vi "Мажор +++.vi"() -> ()   [LabVIEW 2017]
panel:
  in  "Задержка, мс":u32(knob) scale=0.0..10000.0
  in  "?":bool
  in  "Запуск программы":bool
  out "String":string
  in  "Искуственный ввод ошибки":T1(tab)
  in  "Номер элемента со второй ошибкой":i32
  in  "Номер элемента с первой ошибкой":i32
  in  "Номер элемента с третьей ошибкой":i32
  in  "Первый пакет с ошибкой":i32
  in  "Второй пакет с ошибкой":i32
  out "Первый элемент с ошибкой":i32
  out "Второй элемент с ошибкой":i32=16
  out "Третий элемент с ошибкой":i32
  out "Ошибка":bool
  out "Количество  ошибок":i32
  out "Сообщение выдаваемое получателю":dbl[](array[numeric])
  out "Сообщение на выходе канала":dbl[](array[numeric])
  out "2-х массив передаваемых данных":dbl[][](array[numeric])
  out "Массив данных поступающий в канал связи":dbl[](array[numeric])
  in  "Количество передаваемых копий":i32=5
  out "Сообщение источника":dbl[](array[numeric])
  in  "Количество генерируемых данных":i32=16
  # "Мажоритарное резервирование"
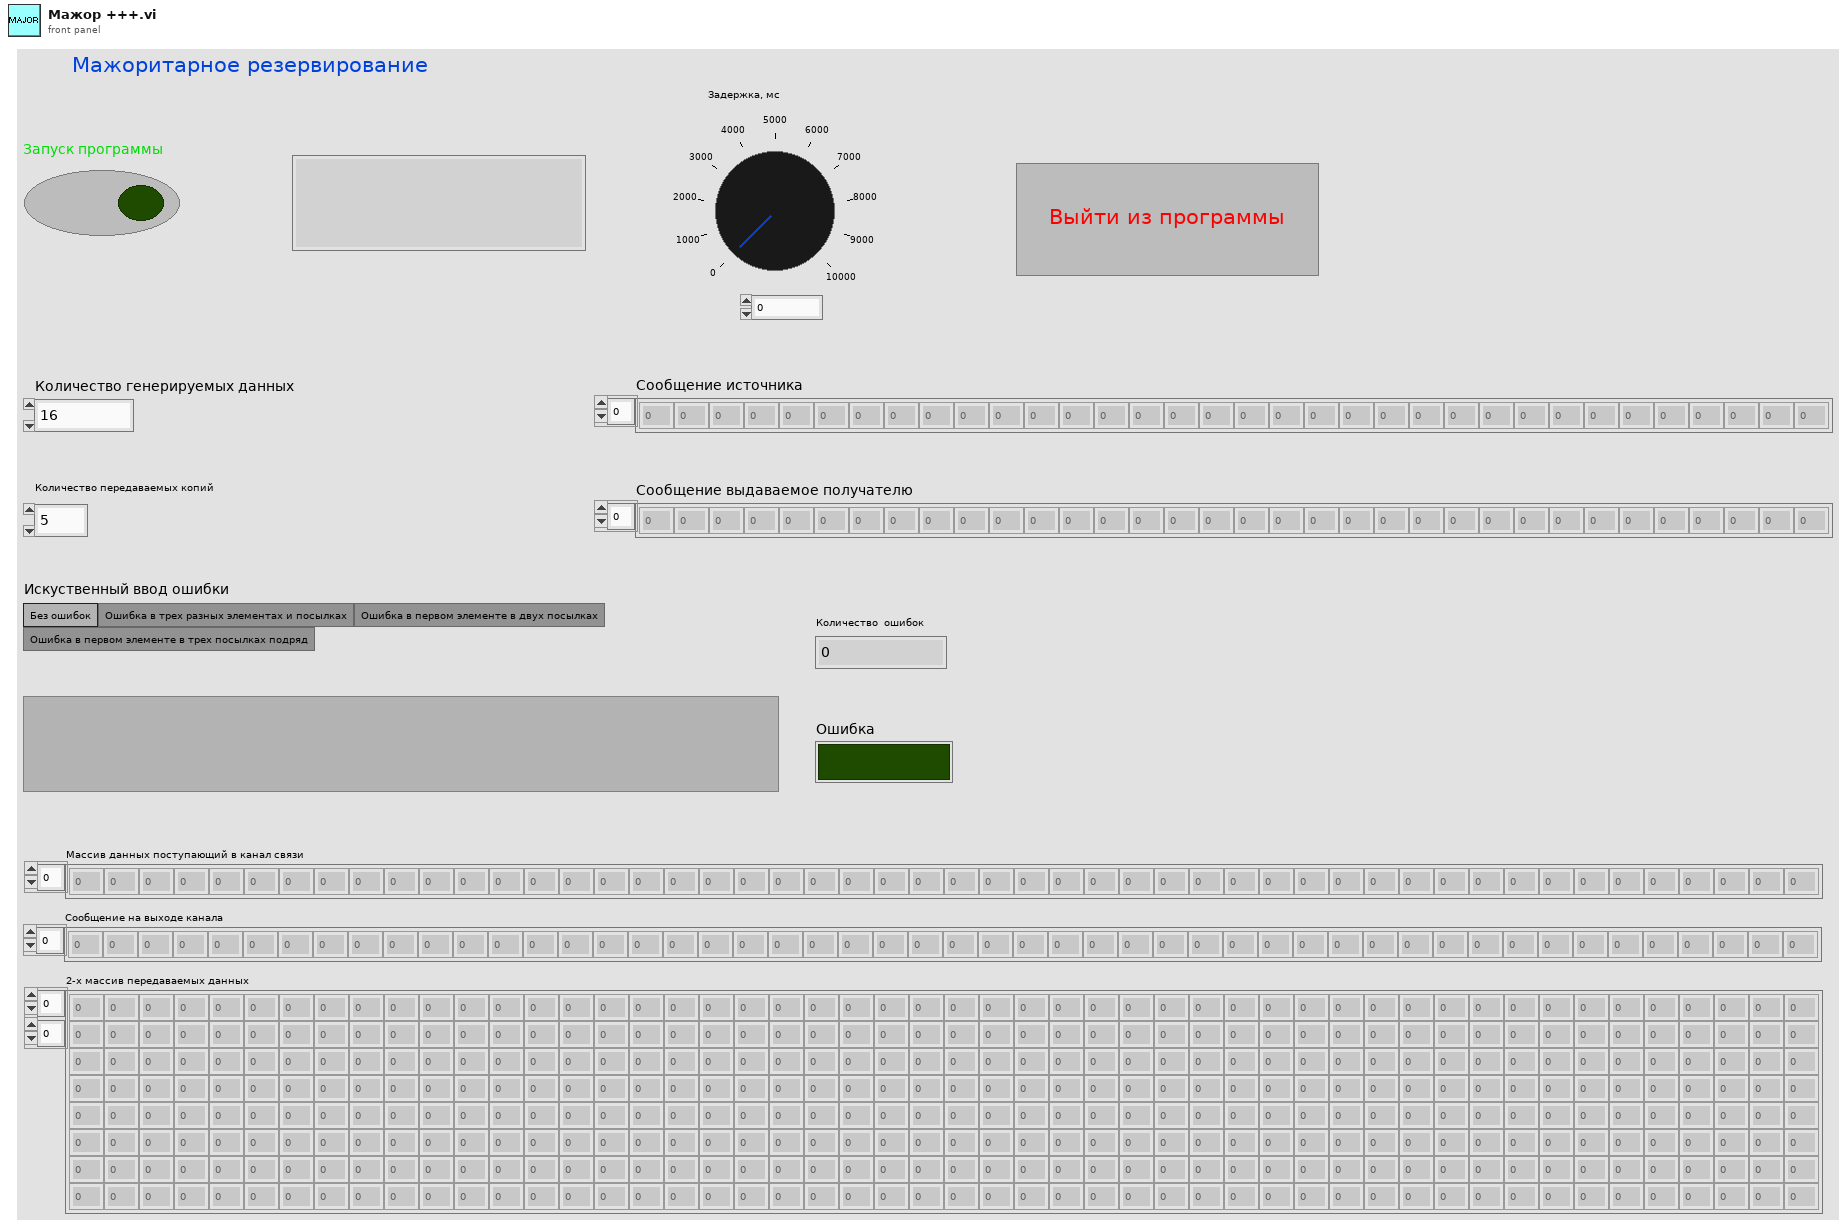
[diagram p1: front panel]
types:
  T1 = enum32{"Без ошибок", "Ошибка в трех разных элементах и посылках", "Ошибка в первом элементе в двух посылках", "Ошибка в первом элементе в трех посылках подряд"}
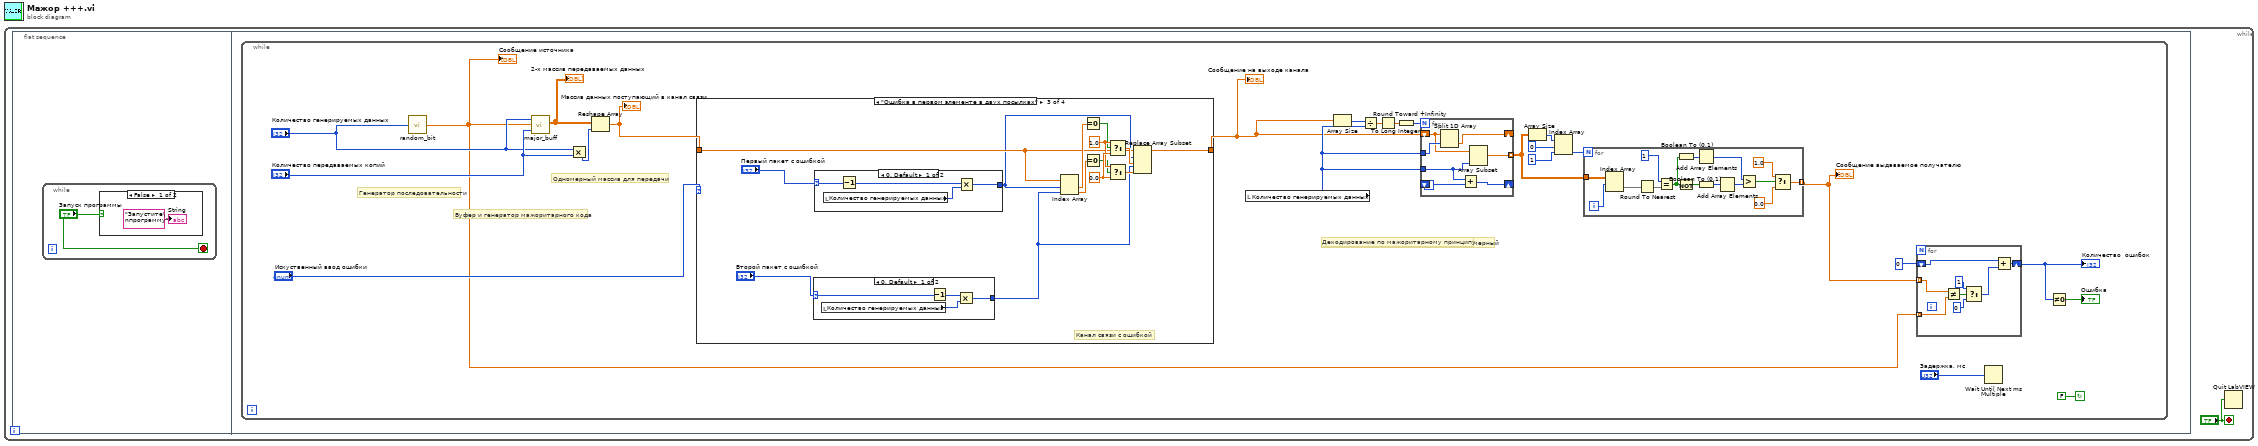
[diagram p0: block diagram]
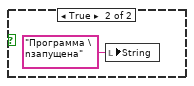
[diagram p2: hidden frame]
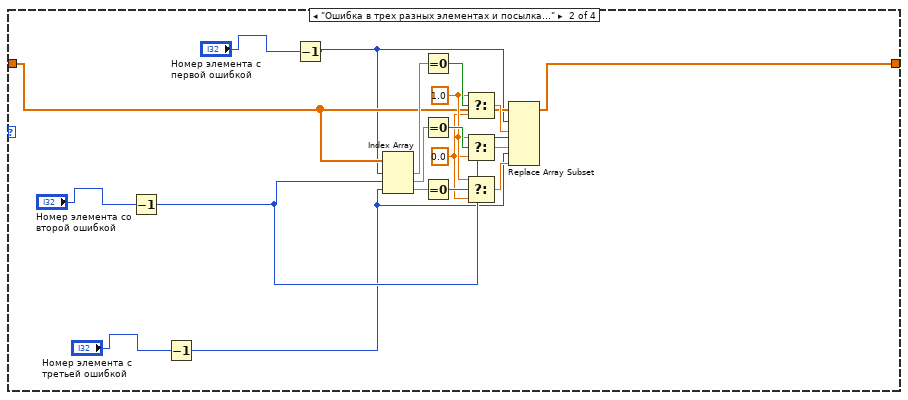
[diagram p4: hidden frame]
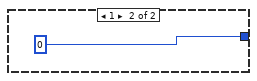
[diagram p5: hidden frame]
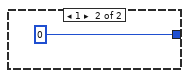
[diagram p6: hidden frame]
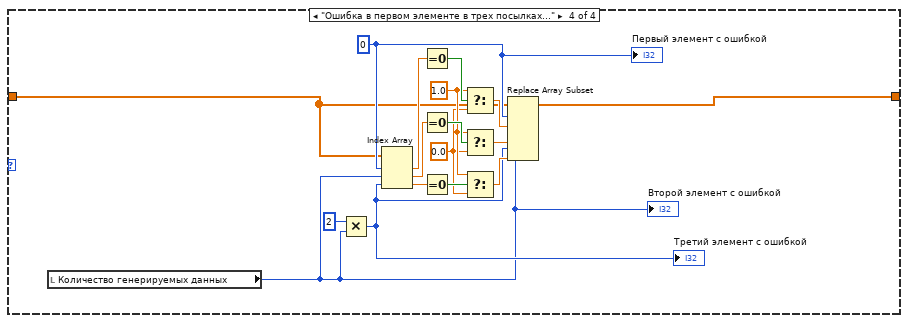
[diagram p7: hidden frame]
diagram:
  n1 = while {
    stop <- "?" stop-if-true
    n2 = flat-sequence {
      frame #0 {
        n3 = while {
          stop <- "Запуск программы" stop-if-true
          n4 = case shown="False" "Запуск программы" {
            frame False {
              "String" <- "Запустите\nпрограмму"
            }
            frame True {
              n5 = local write "String"("Программа \nзапущена") -> ()
            }
          }
        }
      }
      frame #1 {
        n6 = while {
          stop <- FALSE continue-if-true
          # "Канал связи с ошибкой"
          # "Одномерный массив для передачи"
          # "Преобразование одномерного массива в двумерный"
          # "Декодирование по мажоритарному принципу"
          # "Буфер и генератор мажоритарного кода"
          # "Генератор последовательности"
          n7 = call "random_bit.vi"("Количество бит"="Количество генерируемых данных") -> ("Биты на выходе 1"=w14:dbl[])
          "Сообщение источника" <- w14
          n8 = call "major_buff.vi"("Кол-во копий"="Количество передаваемых копий", "Размер окна"="Количество генерируемых данных", "Биты на выходе 1"=w14) -> ("Подготовленный к отправке мажоритарный код"=w17:dbl[][])  [unwired: 1 out]
          "2-х массив передаваемых данных" <- w17
          n9 = Multiply(x="Количество генерируемых данных", y="Количество передаваемых копий") -> (x*y=w25:i32)
          n10 = Reshape Array(w17, w25) -> (w11:dbl[])
          "Массив данных поступающий в канал связи" <- w11
          n11 = case shown="\"Ошибка в первом элементе в двух посылках\"" "Искуственный ввод ошибки" {
            tunnel: w11 -> [w44 w52 w69 w89]
            tunnel: [w44 w51 w68 w88] -> w10
            frame "Без ошибок", Default {
            }
            frame "Ошибка в трех разных элементах и посылках" {
              w57 = 1.0
              w56 = 0.0
              n12 = Decrement(x="Номер элемента со второй ошибкой") -> (x-1=w47:i32)
              n13 = Decrement(x="Номер элемента с третьей ошибкой") -> (x-1=w45:i32)
              n14 = Decrement(x="Номер элемента с первой ошибкой") -> (x-1=w50:i32)
              n15 = Index Array(array=w52, index #1=w50, index #2=w47, index #3=w45) -> (element #1=w63:dbl, element #2=w62:dbl, element #3=w61:dbl)
              n16 = Equal To 0?(x=w63) -> (x = 0?=w60:bool)
              n17 = Equal To 0?(x=w62) -> (x = 0?=w59:bool)
              n18 = Equal To 0?(x=w61) -> (x = 0?=w58:bool)
              n19 = Select(t=w57, s=w60, f=w56) -> (s? t:f=w55:dbl)
              n20 = Select(t=w57, s=w59, f=w56) -> (s? t:f=w54:dbl)
              n21 = Select(t=w57, s=w58, f=w56) -> (s? t:f=w53:dbl)
              n22 = Replace Array Subset(array=w52, new element #1=w55, index #1=w50, new element #2=w54, index #2=w47, new element #3=w53, index #3=w45) -> (w51:dbl[])
            }
            frame "Ошибка в первом элементе в двух посылках" {
              w74 = 1.0
              w75 = 0.0
              n23 = case shown="0, Default" "Второй пакет с ошибкой" {
                selector: "Второй пакет с ошибкой" -> [w78 _]
                tunnel: [w81 0] -> w64
                frame 0, Default {
                  n24 = local read "Количество генерируемых данных"() -> (w80:i32)
                  n25 = Decrement(x=w78) -> (x-1=w79:i32)
                  n26 = Multiply(x=w79, y=w80) -> (x*y=w81:i32)
                }
                frame 1 {
                }
              }
              n27 = case shown="0, Default" "Первый пакет с ошибкой" {
                selector: "Первый пакет с ошибкой" -> [w83 _]
                tunnel: [w86 0] -> w66
                frame 0, Default {
                  n28 = local read "Количество генерируемых данных"() -> (w85:i32)
                  n29 = Decrement(x=w83) -> (x-1=w84:i32)
                  n30 = Multiply(x=w84, y=w85) -> (x*y=w86:i32)
                }
                frame 1 {
                }
              }
              n31 = Index Array(array=w69, index #1=w66, index #2=w64) -> (element #1=w70:dbl, element #2=w71:dbl)
              n32 = Equal To 0?(x=w70) -> (x = 0?=w72:bool)
              n33 = Equal To 0?(x=w71) -> (x = 0?=w73:bool)
              n34 = Select(t=w74, s=w72, f=w75) -> (s? t:f=w76:dbl)
              n35 = Select(t=w74, s=w73, f=w75) -> (s? t:f=w77:dbl)
              n36 = Replace Array Subset(array=w69, new element #1=w76, index #1=w66, new element #2=w77, index #2=w64) -> (w68:dbl[])
            }
            frame "Ошибка в первом элементе в трех посылках подряд" {
              w98 = 1.0
              w97 = 0.0
              w94 = 0
              n37 = local read "Количество генерируемых данных"() -> (w90:i32)
              "Второй элемент с ошибкой" <- w90
              n38 = Multiply(x=2, y=w90) -> (x*y=w92:i32)
              "Третий элемент с ошибкой" <- w92
              n39 = Index Array(array=w89, index #1=w94, index #2=w90, index #3=w92) -> (element #1=w104:dbl, element #2=w103:dbl, element #3=w102:dbl)
              n40 = Equal To 0?(x=w104) -> (x = 0?=w101:bool)
              n41 = Equal To 0?(x=w103) -> (x = 0?=w100:bool)
              n42 = Equal To 0?(x=w102) -> (x = 0?=w99:bool)
              n43 = Select(t=w98, s=w101, f=w97) -> (s? t:f=w96:dbl)
              n44 = Select(t=w98, s=w100, f=w97) -> (s? t:f=w95:dbl)
              n45 = Select(t=w98, s=w99, f=w97) -> (s? t:f=w93:dbl)
              n46 = Replace Array Subset(array=w89, new element #1=w96, index #1=w94, new element #2=w95, index #2=w90, new element #3=w93, index #3=w92) -> (w88:dbl[])
              "Первый элемент с ошибкой" <- w94
            }
          }
          "Сообщение на выходе канала" <- w10
          n47 = local read "Количество генерируемых данных"() -> (w16:i32)
          n48 = Array Size(array=w10) -> (size(s)=w21:i32)
          n49 = Divide(x=w21, y=w16) -> (x/y=w20:dbl)
          n50 = Round Toward +Infinity(x=w20) -> (ceil(x): smallest int >= x=w19:dbl)
          n51 = To Long Integer(number=w19) -> (32bit integer=w18:i32)
          n52 = for {
            N: w18 -> [_]
            shift-right: [w119] -> _
            shift-left: w10 -> [w117]
            tunnel: w16 -> [w118]
            shift-right: [w115] -> _
            shift-left: _ -> [w114]
            tunnel: w16 -> [w116]
            tunnel: [w113] -> w9 mode=indexing
            n53 = Split 1D Array(array=w117, index=w118) -> (second subarray=w119:dbl[])  [unwired: 1 out]
            n54 = Add(x=w116, y=w114) -> (x+y=w115:i32)
            n55 = Array Subset(array=w117, length=w116) -> (w113:dbl[])  [unwired: 1 in]
          }
          n56 = Array Size(array=w9) -> (size(s)=w24:i32[])
          n57 = Index Array(array=w24, index #1=0 ("index"), index #2=1 ("index")) -> (element #2=w7:i32)  [unwired: 1 out]
          n58 = for {
            N: w7 -> [_]
            tunnel: w9 -> [w43]
            tunnel: [w31] -> w8 mode=indexing
            i -> [w29]
            n59 = Index Array(array=w43, index (col)=w29) -> (element=w30:dbl[])  [unwired: 1 in]
            n60 = Round To Nearest(number=w30) -> (nearest integer value=w34:dbl[])
            n61 = Equal?(x=1, y=w34) -> (x = y?=w36:bool[])
            n62 = Boolean To (0,1)(Boolean=w36) -> (0, 1=w33:i16[])
            n63 = Not(x=w36) -> (.not. x?=w37:bool[])
            n64 = Add Array Elements(numeric array=w33) -> (sum=w39:i16)
            n65 = Boolean To (0,1)(Boolean=w37) -> (0, 1=w32:i16[])
            n66 = Add Array Elements(numeric array=w32) -> (sum=w38:i16)
            n67 = Greater?(x=w39, y=w38) -> (0:w42:bool)
            n68 = Select(t=1.0, s=w42, f=0.0) -> (s? t:f=w31:dbl)
          }
          "Сообщение выдаваемое получателю" <- w8
          n69 = for {
            tunnel: w8 -> [w112] mode=indexing
            tunnel: w14 -> [w111] mode=indexing
            shift-right: [w106] -> w12
            shift-left: 0 -> [w105]
            n70 = Not Equal?(x=w112, y=w111) -> (x != y?=w107:bool)
            n71 = Select(t=1, s=w107, f=0) -> (s? t:f=w108:i32)
            n72 = Add(x=w105, y=w108) -> (x+y=w106:i32)
          }
          "Количество  ошибок" <- w12
          n73 = Wait Until Next ms Multiple(millisecond multiple="Задержка, мс") -> ()  [unwired: 1 out]
          n74 = Not Equal To 0?(x=w12) -> (x != 0?=→"Ошибка":bool)
        }
      }
    }
    n75 = Quit LabVIEW(quit? (T)="?") -> ()
  }
